vi "Temperature serial v2.vi"(0 "Command String":string, 5 "com port":refnum<visa-resource-name>) -> (3 "ID":dbl, 4 "T1":dbl, 6 "T2":dbl, 8 "T3":dbl, 10 "T4":dbl, 13 "error":bool, 15 "out array":i32[](array[numeric]))   [LabVIEW 2017]
uses:
  <vilib>/Platform/TimedLoop/XDataNode/timing_clust.ctl
  <vilib>/Platform/TimedLoop/XDataNode/nitl_modes.ctl
  <vilib>/Platform/TimedLoop/XDataNode/wakeup.ctl
  <vilib>/Instr/_visa.llb/VISA Configure Serial Port (Instr).vi
  <vilib>/platform/TimedLoop/XDataNode/XDataNode.xnode
  <vilib>/Platform/TimedLoop/XDataNode/XDNodeRunTimeDep.lvlib
panel:
  out "LOOP":bool
  in  "Array - String":string[](array[string])
  out "end of data (#)":bool
  out "data bytes read":dbl
  out "data string":string
  out "read buffer":string
  out "error out":errorcluster
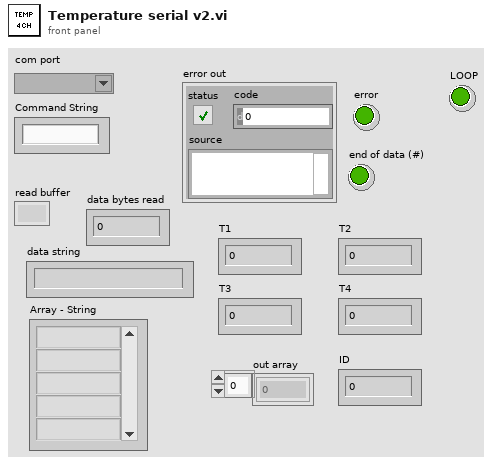
[diagram p1: front panel]
types:
  T1 = typedef "XDNodeRunTimeDep.lvlib/timing_clust.ctl" = cluster{"Expected End [f-1]":u64, "Actual End [f-1]":u64, "Finished Late? [f-1]":bool, "Expected End [i-1]":u64, "Actual End [i-1]":u64, "Finished Late? [i-1]":bool, "Expected Start [i]":u64, "Actual Start [i]":u64, "Expected Start [f]":u64, "Actual Start [f]":u64, "Source Name":string, "Structure Name":string, "Period":i64, "Deadline":i64, "Offset":i64, "Start":i64, "Priority":i32, "Timeout":i32, "Mode":T2, "Wakeup Reason":T3, "Error":errorcluster, "Source Type":string, "Secondary Source Type":string, "Global End Time":u64, "Global Start Time":u64, "Frame Duration":u64, "Iteration Duration":u64, "Assigned CPU":i32, "I/O Scan Engine Mode":u32}
  T2 = typedef "XDNodeRunTimeDep.lvlib/nitl_modes.ctl" = enum32{"No Change", "Process missed periods, maintain original phase", "Discard missed periods, maintain original phase", "Process missed periods, ignore original phase", "Discard missed periods, ignore original phase"}
  T3 = typedef "XDNodeRunTimeDep.lvlib/wakeup.ctl" = enum32{"Normal", "Aborted", "Asynchronous wakeup", "Timing source error", "Timed loop error", "Timeout"}
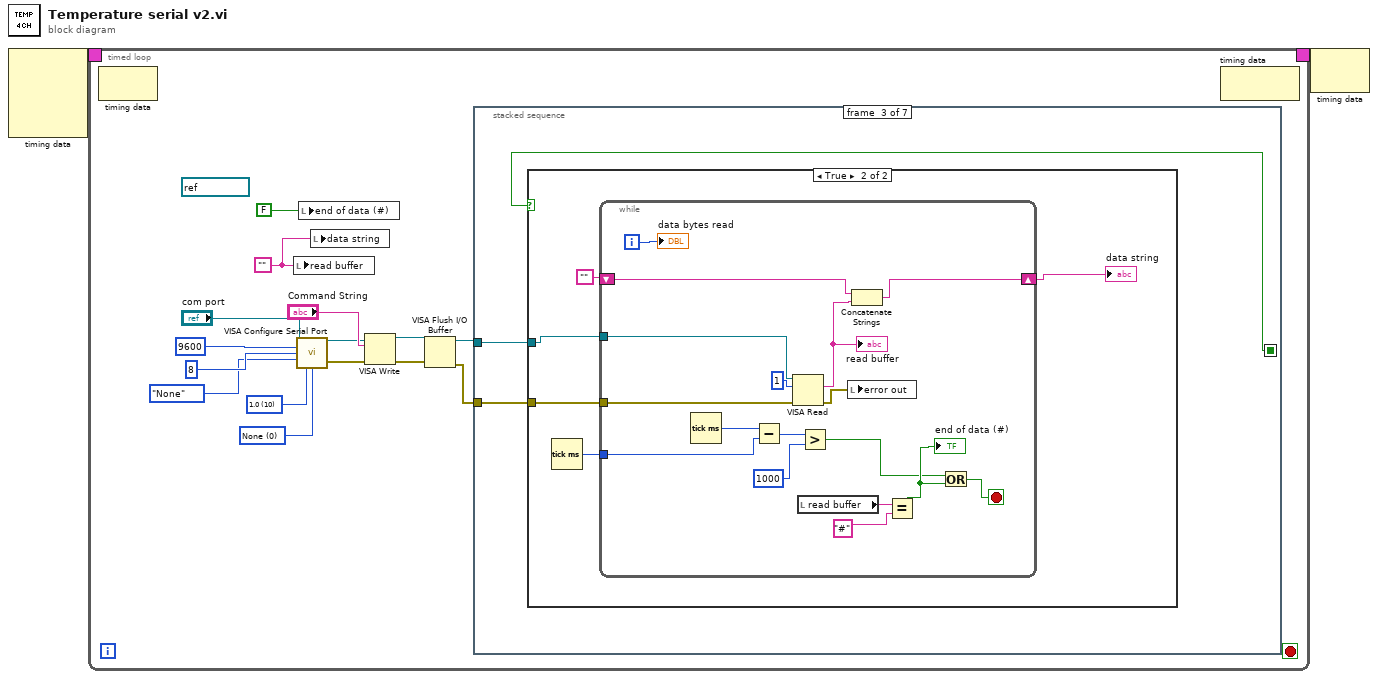
[diagram p0: block diagram]
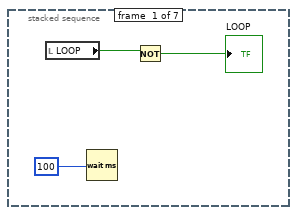
[diagram p2: hidden frame]
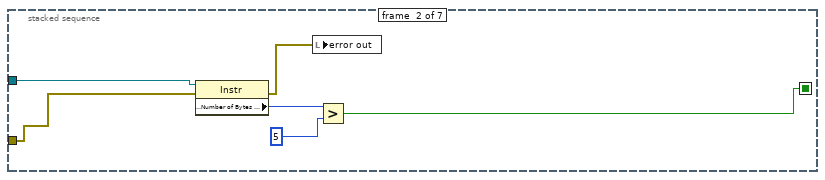
[diagram p3: hidden frame]
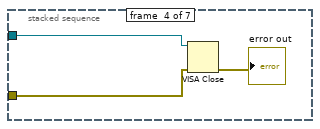
[diagram p5: hidden frame]
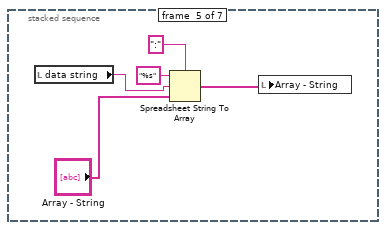
[diagram p6: hidden frame]
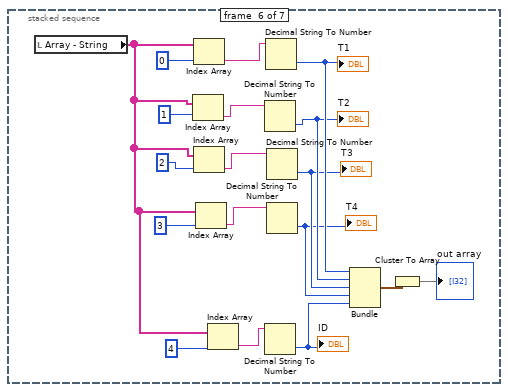
[diagram p7: hidden frame]
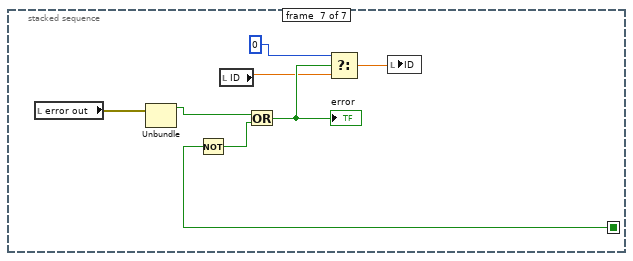
[diagram p8: hidden frame]
diagram:
  n1 = node-c288() -> (w2:T1)  [unwired: 4 in]
  n2 = timed-loop {
    timing: w2 -> [_]
    timing-out: [_] -> w1
    stop <- _ stop-if-true
    w3 = ""
    w13 = u16 0 items=["None", "XON/XOFF", "RTS/CTS", "XON/XOFF & RTS/CTS", "DTR/DSR", "XON/XOFF & DTR/DSR"] ("flow control (0:none)")
    w14 = u16 10 items=["1.0"=10, "1.5"=15, "2.0"=20] ("stop bits (10: 1 bit)")
    (unwired) refnum<visa-resource-name> "COM10" ("VISA resource name")
    n3 = node-c288() -> ()  [unwired: 1 in, 1 out]
    n4 = local write "read buffer"(w3) -> ()
    n5 = call-poly "VISA Configure Serial Port"("VISA resource name"="com port", "baud rate (9600)"=u32 9600, "data bits (8)"=u16 8, "parity (0:none)"=enum16{"None", "Odd", "Even", "Mark", "Space"}."None", "stop bits (10: 1 bit)"=w14, "flow control (0:none)"=w13) -> ("VISA resource name out"=w6:refnum<visa-resource-name>, "error out"=w5:errorcluster)  [unwired: 8 in]
    n6 = local write "end of data (#)"(FALSE) -> ()
    n7 = local write "data string"(w3) -> ()
    n8 = VISA Write(VISA resource name=w6, write buffer="Command String", error in (no error)=w5) -> (VISA resource name out=w11:refnum<visa-resource-name>, error out=w10:errorcluster)  [unwired: 1 out]
    n9 = VISA Flush I/O Buffer(VISA resource name=w11, error in (no error)=w10) -> (VISA resource name out=w9:refnum<visa-resource-name>, error out=w8:errorcluster)  [unwired: 1 in]
    n10 = stacked-sequence {
      seq-local: [_ w22 _ _ _ _ _] -> [_ _ w27 _ _ _ w83]
      tunnel: w9 -> [_ w26 w29 w54 _ _ _]
      tunnel: w8 -> [_ w25 w28 w53 _ _ _]
      frame #0 {
        n11 = local read "LOOP"() -> (w19:bool)
        n12 = Wait (ms)(milliseconds to wait=100) -> ()  [unwired: 1 out]
        n13 = Not(x=w19) -> (.not. x?=→"LOOP":bool)
      }
      frame #1 {
        n14 = property class="Instr"(reference=w26, error in=w25) -> (error out=w21:errorcluster, "Serial Settings:Number of Bytes at Serial Port"=w24:u32)  [unwired: 1 out]
        n15 = local write "error out"(w21) -> ()
        n16 = Greater?(x=w24, y=5) -> (0:w22:bool)
      }
      frame #2 {
        n17 = case shown="True" w27 {
          tunnel: w29 -> [_ w34]
          tunnel: w28 -> [_ w33]
          frame False {
          }
          frame True {
            n18 = Tick Count (ms)() -> (millisecond timer value=w30:u32)
            n19 = while {
              tunnel: w34 -> [w46]
              tunnel: w33 -> [w45]
              shift-right: [w44] -> w32
              shift-left: "" -> [w43]
              tunnel: w30 -> [w40]
              i -> [w47]
              stop <- w35 stop-if-true
              n20 = Tick Count (ms)() -> (millisecond timer value=w41:u32)
              n21 = Subtract(x=w41, y=w40) -> (x-y=w39:u32)
              n22 = VISA Read(VISA resource name=w46, byte count=u32 1, error in (no error)=w45) -> (read buffer=w48:string, error out=w42:errorcluster)  [unwired: 2 out]
              "read buffer" <- w48
              n23 = local read "read buffer"() -> (w50:string)
              n24 = Greater?(x=w39, y=u32 1000) -> (0:w36:bool)
              n25 = local write "error out"(w42) -> ()
              n26 = Concatenate Strings(w43, w48) -> (w44:string)
              n27 = Equal?(x=w50, y="#") -> (x = y?=w37:bool)
              "end of data (#)" <- w37
              n28 = Or(x=w36, y=w37) -> (x .or. y?=w35:bool)
              "data bytes read" <- w47
            }
            "data string" <- w32
          }
        }
      }
      frame #3 {
        n29 = VISA Close(VISA resource name=w54, error in (no error)=w53) -> (error out=→"error out":errorcluster)
      }
      frame #4 {
        n30 = local read "data string"() -> (w57:string)
        n31 = Spreadsheet String To Array(delimiter (Tab)=":", format string="%s", spreadsheet string=w57, array type (2D Dbl)="Array - String") -> (array=w55:string[])
        n32 = local write "Array - String"(w55) -> ()
      }
      frame #5 {
        n33 = local read "Array - String"() -> (w63:string[])
        n34 = Index Array(array=w63, index=1) -> (element=w72:string)
        n35 = Index Array(array=w63, index=0) -> (element=w76:string)
        n36 = Index Array(array=w63, index=2) -> (element=w71:string)
        n37 = Index Array(array=w63, index=3) -> (element=w70:string)
        n38 = Index Array(array=w63, index=4) -> (element=w61:string)
        n39 = Decimal String To Number(string=w72) -> (number=w68:i32)  [unwired: 2 in, 1 out]
        "T2" <- w68
        n40 = Decimal String To Number(string=w61) -> (number=w60:i32)  [unwired: 2 in, 1 out]
        "ID" <- w60
        n41 = Decimal String To Number(string=w76) -> (number=w69:i32)  [unwired: 2 in, 1 out]
        "T1" <- w69
        n42 = Decimal String To Number(string=w71) -> (number=w67:i32)  [unwired: 2 in, 1 out]
        "T3" <- w67
        n43 = Decimal String To Number(string=w70) -> (number=w66:i32)  [unwired: 2 in, 1 out]
        "T4" <- w66
        n44 = Bundle(w69, w68, w67, w66, w60) -> (w65:cluster{i32, i32, i32, i32, i32})  [unwired: 1 in]
        n45 = Cluster To Array(cluster=w65) -> (array=→"out array":i32[])
      }
      frame #6 {
        n46 = local read "error out"() -> (w85:errorcluster)
        n47 = Unbundle(w85) -> ("status"=w84:bool)  [unwired: 2 out]
        n48 = Not(x=w83) -> (.not. x?=w82:bool)
        n49 = local read "ID"() -> (w78:dbl)
        n50 = Or(x=w84, y=w82) -> (x .or. y?=w81:bool)
        "error" <- w81
        n51 = Select(t=0, s=w81, f=w78) -> (s? t:f=w79:dbl)
        n52 = local write "ID"(w79) -> ()
      }
    }
    n53 = node-c288() -> ()  [unwired: 1 in, 1 out]
  }
  n54 = node-c288(w1) -> ()  [unwired: 1 out]
